vi "Channel_Names_and_indicies.vi"(2 "All Active Channels":bool, 3 "Desired Ch Names":string[](array[string])) -> (0 "Indicies":i32[](array[numeric]), 1 "Active Ch names":string[](array[string]))   [LabVIEW 2010]
uses:
  ADAM_Global.vi
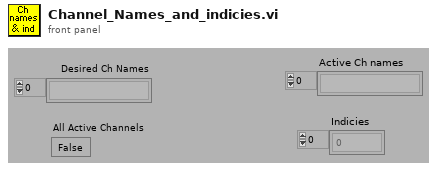
[diagram p1: front panel]
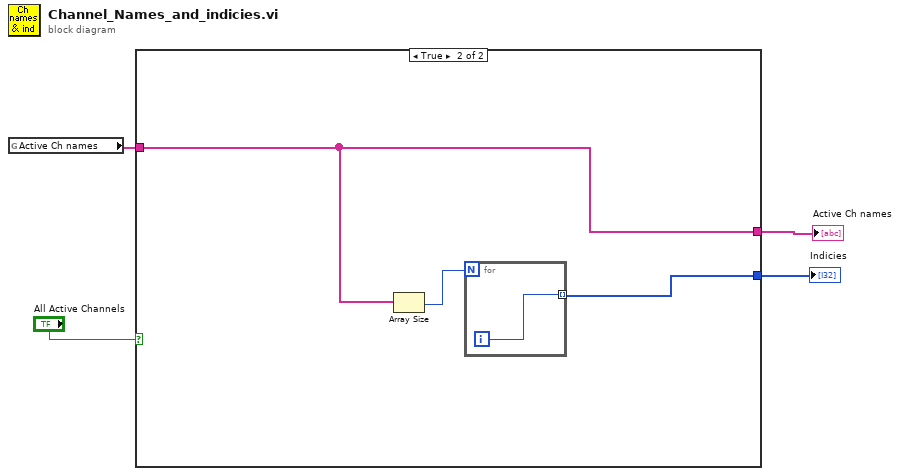
[diagram p0: block diagram]
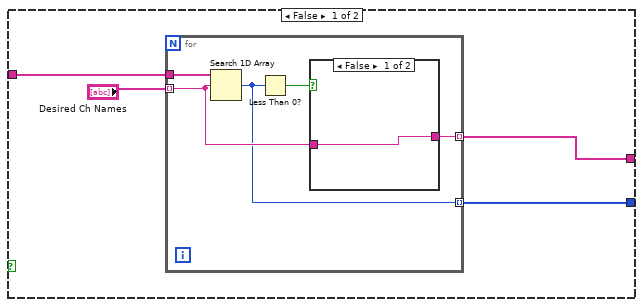
[diagram p2: hidden frame]
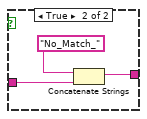
[diagram p3: hidden frame]
diagram:
  n1 = global read "ADAM_Global.vi" "Active Ch names"() -> (w3:string[])
  n2 = case shown="True" "All Active Channels" {
    tunnel: w3 -> [w8 w19]
    tunnel: [w5 w19] -> w2
    tunnel: [w6 w18] -> w1
    frame False {
      n3 = for {
        tunnel: "Desired Ch Names" -> [w12] mode=indexing
        tunnel: w8 -> [w11]
        tunnel: [w10] -> w6 mode=indexing
        tunnel: [w9] -> w5 mode=indexing
        n4 = Search 1D Array(1D array=w11, element=w12) -> (index of element=w10:i32)  [unwired: 1 out]
        n5 = Less Than 0?(x=w10) -> (x < 0?=w13:bool)
        n6 = case shown="False" w13 {
          tunnel: w12 -> [w14 w17]
          tunnel: [w14 w15] -> w9
          frame False {
          }
          frame True {
            n7 = Concatenate Strings("No_Match_" ("string"), w17) -> (w15:string)
          }
        }
      }
    }
    frame True {
      n8 = Array Size(array=w19) -> (size(s)=w20:i32)
      n9 = for {
        N: w20 -> [_]
        tunnel: [w21] -> w18 mode=indexing
        i -> [w21]
      }
    }
  }
  "Active Ch names" <- w2
  "Indicies" <- w1
